vi "FTW-Test-SQLite-JSON.vi"() -> (0 "Test Result":errorcluster)   [LabVIEW 2014]
uses:
  src/core/database/core/FTW-SQLite-Core-PrepareStatement.vi
  src/core/error/FTW-ERR-Assert-DeveloperError.vi
  src/core/error/FTW-ERR-StatusOK.vi
  src/core/database/core/FTW-SQLite-Core-QueryDebug.vi
  src/core/time/FTW-Time-RelativeTimer.vi
  lib/FTW-LibraryFilepath.vi
  src/core/error/FTW-ERR-ThrowError.vi
  src/core/error/FTW-ERR-ThrowGenericError.vi
  src/core/error/FTW-ERR-CallChain.vi
  src/core/string/FTW-STR-ReplaceWhitespace.vi
  src/core/database/core/FTW-SQLite-Core-LibraryReturnValue.vi
  src/core/database/FTW-SQLite-Fetch/FTW-SQLite-Fetch.xnode
  src/core/database/core/FTW-SQLite-Core-Structure.ctl
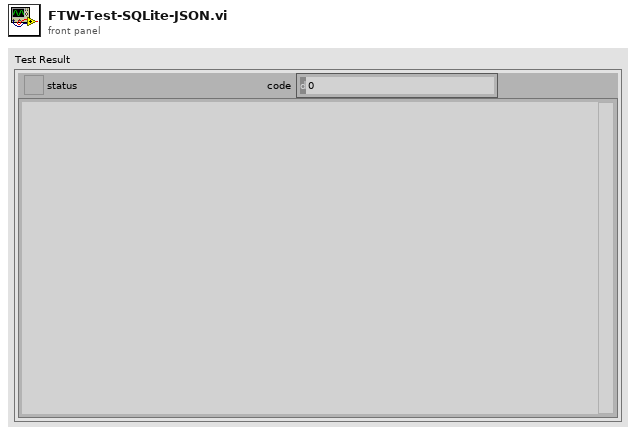
[diagram p1: front panel]
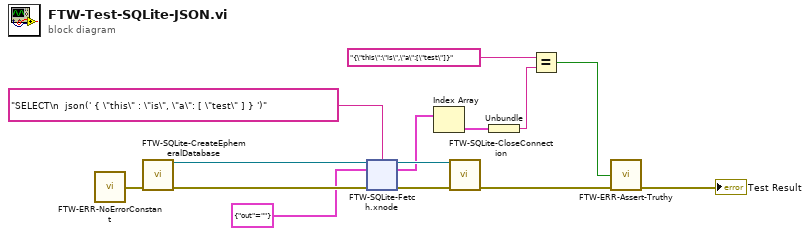
[diagram p0: block diagram]
diagram:
  n1 = call "FTW-ERR-NoErrorConstant.vi"() -> ("no error"=w14:errorcluster)
  n2 = call "FTW-SQLite-CreateEphemeralDatabase.vi"("error in"=w14) -> ("SQLite Connection"=w10:refnum<data-value>, "error out"=w9:errorcluster)  [unwired: 13 in]
  n3 = xnode "FTW-SQLite-Fetch.xnode"("SQLite Connection"=w10, "SQL Script"="SELECT\n  json(' { \"this\" : \"is\", \"a\": [ \"test\" ] } ')", "Row Datatype"=cluster{"out":string} {"out"=""}, "error in"=w9) -> ("SQLite Connection out"=w12:refnum<data-value>, "Result Set"=w7:cluster{"out":string}[], "error out"=w11:errorcluster)  [unwired: 1 out]
  n4 = Index Array(array=w7) -> (element=w6:cluster{"out":string})  [unwired: 1 in]
  n5 = call "FTW-SQLite-CloseConnection.vi"("SQLite Connection"=w12, "error in"=w11) -> ("error out"=w2:errorcluster)  [unwired: 13 in]
  n6 = Unbundle(w6) -> ("out"=w4:string)
  n7 = Equal?(x="{\"this\":\"is\",\"a\":[\"test\"]}", y=w4) -> (x = y?=w3:bool)
  n8 = call "FTW-ERR-Assert-Truthy.vi"("Expected Truthy"=w3, "error in"=w2) -> ("error out"=→"Test Result":errorcluster)  [unwired: 13 in]
